vi "Error Register.vi"(7 "Throw Up?":bool, 8 "error in (no error)":errorcluster, 9 "Specifics":string, 10 "Context":T1 {"name" items=["Method Name", "Parameter Name", "VI Name", "Control Name", "Proxy Dll Path", "Project Library Name"]}, 11 "Error Number":T3 items=["ERR_NOERROR"=0, "ERR_ACCESS_OUTPUTFOLDER"=1, "ERR_INVALID_LIBRARYNAME"=2, "ERR_CREATE_VIWRAPPER"=3, "ERR_UNKNOWN"=201, "ERR_BAD_ARGUMENT"=202, "ERR_URL_NOTFOUND_BADWSDL"=203, "ERR_BADLYFORMATTEDURL"=204, "ERR_BADHOSTNAME"=205, "ERR_BADDIRECTORY"=206, "ERR_UNAUTHORIZEDACCESS"=207, "ERR_CREATELIBRARY"=208, "ERR_COMPILEERROR"=209]) -> (0 "error out":errorcluster)   [LabVIEW 2020, in "WebServiceImporter.lvlib" / "Error Handling.lvlib"]
uses:
  <vilib>/Platform/WebService/Error Handling/Error Handling.lvlib
  <vilib>/Platform/WebService/Error Handling/Error/Error Number.ctl
  <vilib>/Platform/WebService/Error Handling/Error/Context.ctl
  <vilib>/Platform/WebService/Error Handling/Error/Context Name.ctl
  <vilib>/Platform/WebService/Error Handling/Error/Error Info.ctl
  <vilib>/Platform/WebService/Error Handling/Error/Operation.ctl
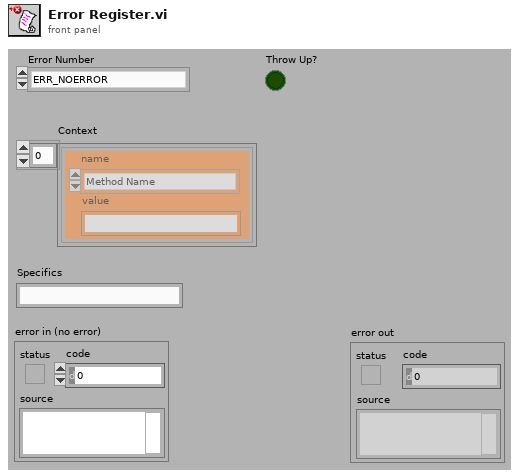
[diagram p1: front panel]
types:
  T1 = typedef "WebServiceImporter.lvlib/Error Handling.lvlib/Context.ctl" = cluster{"name":T2, "value":string}[]
  T2 = typedef "WebServiceImporter.lvlib/Error Handling.lvlib/Context Name.ctl" = u16
  T3 = typedef "WebServiceImporter.lvlib/Error Handling.lvlib/Error Number.ctl" = u16
  T4 = typedef "WebServiceImporter.lvlib/Error Handling.lvlib/Operation.ctl" = enum16{"Get", "Add", "Clear"}
  T5 = typedef "WebServiceImporter.lvlib/Error Handling.lvlib/Error Info.ctl" = cluster{"Specifics":string, "Error Number":T3, "Call Chain":string, "Context":T1}
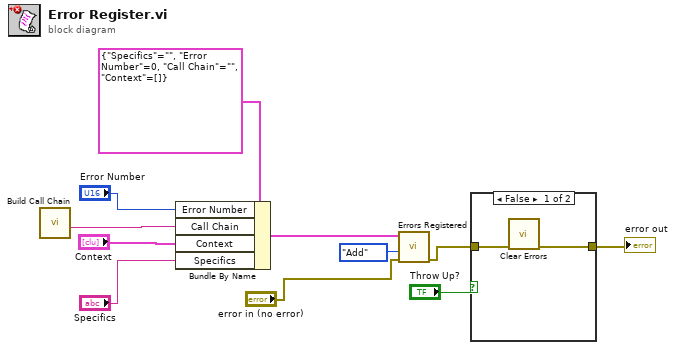
[diagram p0: block diagram]
diagram:
  n1 = call <vilib>:"Build Call Chain.vi"() -> ("Call Chain"=w1:string)  [unwired: 11 in]
  n2 = Bundle By Name(cluster=T5 {"Specifics"="", "Error Number"=0, "Call Chain"="", "Context"=[]} ("Error Info"), "Error Number"="Error Number", "Call Chain"=w1, "Context"="Context", "Specifics"="Specifics") -> (w4:T5)
  n3 = call <vilib>:"Errors Registered.vi"("error in (no error)"="error in (no error)", "Operation"=Operation."Add", "Error Info"=w4) -> ("error out"=w2:errorcluster)  [unwired: 7 in, 1 out]
  n4 = case shown="False" "Throw Up?" {
    tunnel: w2 -> [w13 w14]
    tunnel: [w12 w14] -> w10
    frame False {
      n5 = call <vilib>:"Clear Errors.vi"("error in (no error)"=w13) -> ("error out"=w12:errorcluster)  [unwired: 5 in, 1 out]
    }
    frame True {
    }
  }
  "error out" <- w10
